vi "zadanie1_kol.vi"() -> ()   [LabVIEW 2012]
panel:
  in  "oblliczaj napiêcie || obliczaj natê¿enie":bool
  out "wyniki:":cluster{i32, dbl}[](graph)
  in  "Podaj wartoœæ rezystancji [Om]":dbl
  # "Program przedstawia dzi³anie prawa Ohma\nU¿ytkownik podaje wartoœæ rezystancji, a nastêpnie wybiera czy chce obliczaæ napiêcie \nna podtawie rosn¹cego co 1 od 0 do 100 wartoœci natê¿enia czy chce obliczaæ natêzenie na podstawie rosn¹cego napiêcia\nNastêpnie wyniki przedstawiane œ¹ w formie punktów na poni¿szym wykresie"
  # "prawo Ohma:\nR = U/I\nR - rezystancja\nU - napiêcie\nI - natê¿enie"
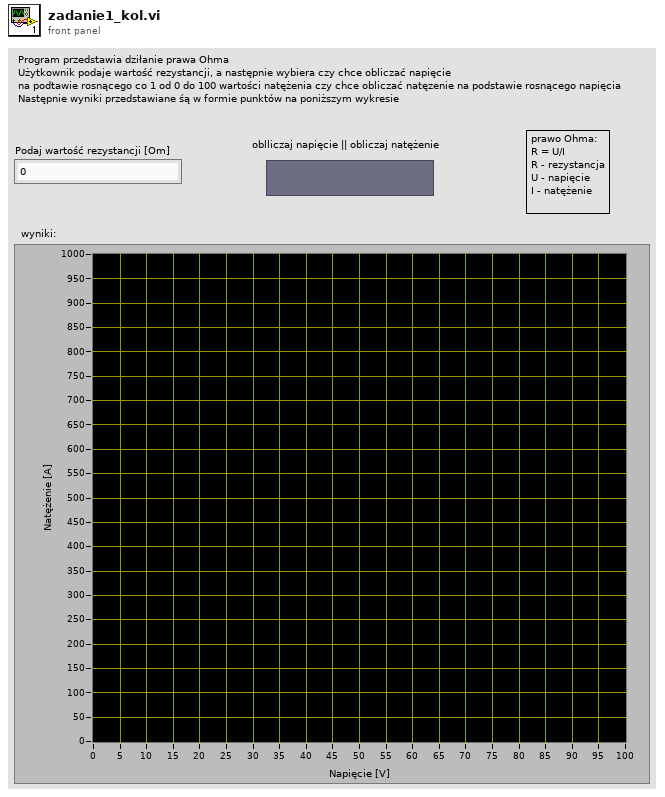
[diagram p1: front panel]
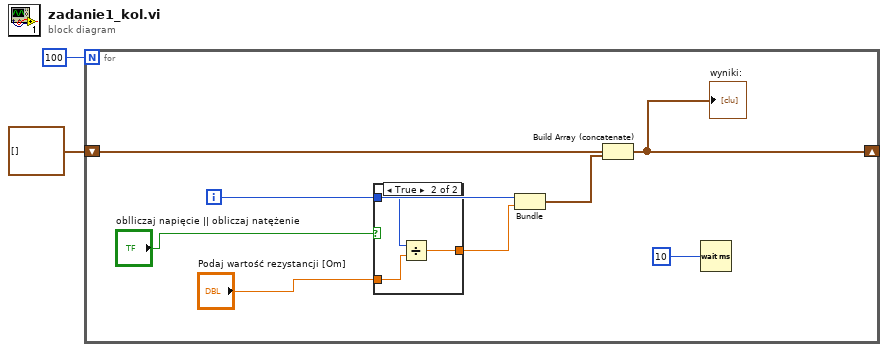
[diagram p0: block diagram]
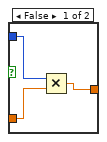
[diagram p2: hidden frame]
diagram:
  n1 = for {
    N: 100 -> [_]
    shift-right: [w8] -> _
    shift-left: cluster{i32, i32}[] [] -> [w7]
    i -> [w6]
    n2 = case shown="True" "oblliczaj napiêcie || obliczaj natê¿enie" {
      tunnel: w6 -> [w12 w16]
      tunnel: "Podaj wartoœæ rezystancji [Om]" -> [w11 w15]
      tunnel: [w13 w14] -> w4
      frame False {
        n3 = Multiply(x=w12, y=w11) -> (x*y=w13:dbl)
      }
      frame True {
        n4 = Divide(x=w16, y=w15) -> (x/y=w14:dbl)
      }
    }
    n5 = Bundle(w6, w4) -> (w9:cluster{i32, dbl})  [unwired: 1 in]
    n6 = Build Array (concatenate)(w7, w9) -> (w8:cluster{i32, dbl}[])
    "wyniki:" <- w8
    n7 = Wait (ms)(milliseconds to wait=10) -> ()  [unwired: 1 out]
  }
